vi "Handshake.vi"(8 "error in (no error)":errorcluster, 9 "Timeout (5000ms)":u32=5000, 11 "OpenSSL in":refnum<class "SSL Server Socket.lvclass">) -> (0 "error out":errorcluster, 3 "OpenSSL out":refnum<class "SSL Server Socket.lvclass">)   [LabVIEW 2013, in "OpenSSL Socket.lvlib" / "SSL Server Socket.lvclass"]
uses:
  SSL Server Socket.lvclass
  Secure Socket/SSL Socket.lvclass/SSL Socket.ctl
  Secure Socket/Read BIO.vi
  SSL_Lib/BIO/BIO.lvclass
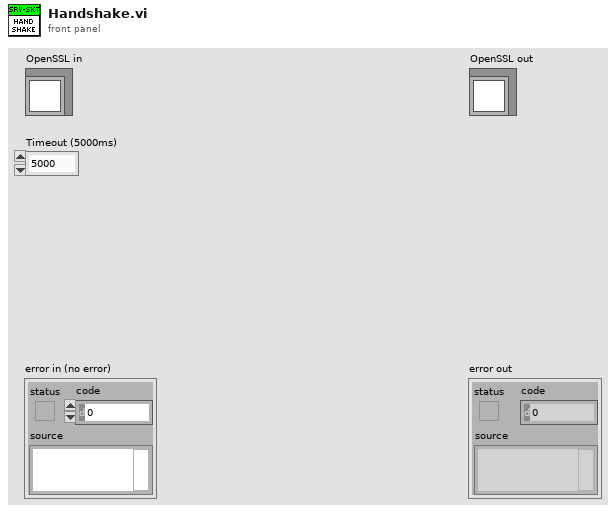
[diagram p1: front panel]
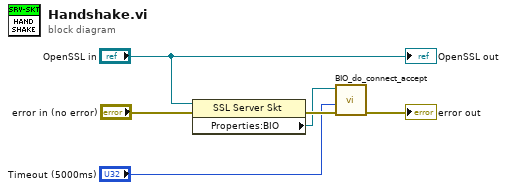
[diagram p0: block diagram]
diagram:
  n1 = property class="SSL Server Skt"(reference="OpenSSL in", error in="error in (no error)") -> (error out=w5:errorcluster, "Properties:BIO"=w4:refnum<class "BIO.lvclass">)  [unwired: 1 out]
  n2 = call "BIO_do_connect_accept.vi"("error in (no error)"=w5, "Timeout (10000ms)"="Timeout (5000ms)", "BIO in"=w4) -> ("error out"=→"error out":errorcluster)  [unwired: 7 in, 1 out]
  "OpenSSL out" <- "OpenSSL in"
